vi "Do Van Der Pauw Calculations.vi"(8 "error in (no error)":errorcluster) -> (0 "error out":errorcluster)   [LabVIEW 2016, in "Hall Effect Library.lvlib"]
uses:
  Hall Effect Library.lvlib
  Global Variables/Hall Effect Data.vi
  Global Variables/Test Settings.vi
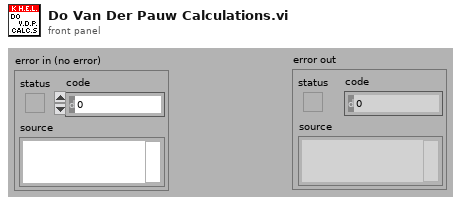
[diagram p1: front panel]
types:
  T1 = cluster{"fA":dbl, "fB":dbl, "QA":dbl, "QB":dbl, "pAvg":dbl, "pA":dbl, "pB":dbl}
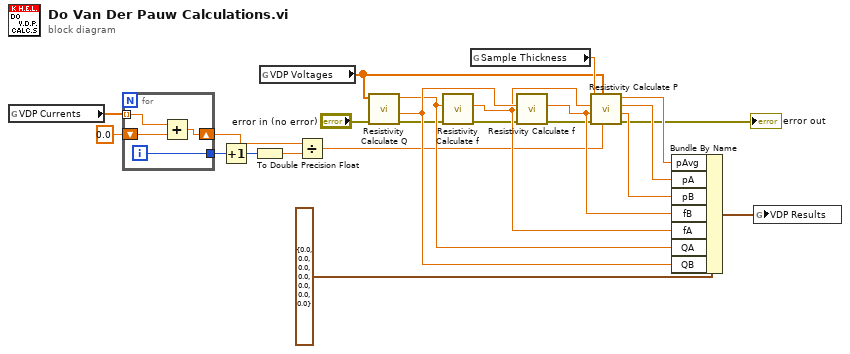
[diagram p0: block diagram]
diagram:
  n1 = global read "Hall Effect Data.vi" "VDP Currents"() -> (w2:dbl[])
  n2 = for {
    tunnel: w2 -> [w27] mode=indexing
    shift-right: [w24] -> w4
    shift-left: 0.0 -> [w26]
    tunnel: [w25] -> w5
    i -> [w25]
    n3 = Add(x=w27, y=w26) -> (x+y=w24:dbl)
  }
  n4 = Increment(x=w5) -> (x+1=w7:i32)
  n5 = To Double Precision Float(number=w7) -> (double precision float=w6:dbl)
  n6 = global read "Hall Effect Data.vi" "VDP Voltages"() -> (w15:dbl[])
  n7 = Divide(x=w4, y=w6) -> (x/y=w1:dbl)
  n8 = call "Resistivity Calculate Q.vi"("error in (no error)"="error in (no error)", "V1-V8 VDP"=w15) -> ("error out"=w14:errorcluster, "QB"=w23:dbl, "QA"=w22:dbl)  [unwired: 7 out]
  n9 = call "Resistivity Calculate f.vi"("error in"=w14, "Q"=w22) -> ("error out"=w13:errorcluster, "f"=w21:dbl)  [unwired: 8 out]
  n10 = global read "Test Settings.vi" "Sample Thickness"() -> (w16:dbl)
  n11 = call "Resistivity Calculate f.vi"("error in"=w13, "Q"=w23) -> ("error out"=w12:errorcluster, "f"=w20:dbl)  [unwired: 8 out]
  n12 = call "Resistivity Calculate P.vi"("Current Level (A)"=w1, "V1-V8 VDP"=w15, "error in (no error)"=w12, "fB"=w20, "fA"=w21, "Thickness (cm)"=w16) -> ("error out"=→"error out":errorcluster, "pB"=w19:dbl, "pA"=w18:dbl, "pAVG"=w17:dbl)  [unwired: 2 out]
  n13 = Bundle By Name(cluster=T1 {"fA"=0.0, "fB"=0.0, "QA"=0.0, "QB"=0.0, "pAvg"=0.0, "pA"=0.0, "pB"=0.0} ("VDP Results"), "pAvg"=w17, "pA"=w18, "pB"=w19, "fB"=w20, "fA"=w21, "QA"=w22, "QB"=w23) -> (w9:T1)
  n14 = global write "Hall Effect Data.vi" "VDP Results"(w9) -> ()
